vi "Process Trainer.vi"() -> ()   [LabVIEW 2019]
uses:
  <vilib>/Modbus/slave/Create Slave Instance (TCP).vi
  <vilib>/Modbus/slave/Modbus Slave.lvclass
panel:
  out "Waveform Graph":sgl[](graph)
  out "Hot water":sgl
  out "L1":sgl
  out "F2":sgl
  out "F1":sgl
  out "T3":sgl
  out "T2":sgl
  out "T1":sgl
  in  "Hot Water Setpoint":sgl(slide) scale=0.0..200.0
  in  "FV4":sgl(slide) scale=0.0..100.0
  in  "FV3":sgl(slide) scale=0.0..100.0
  in  "FV2":sgl(slide) scale=0.0..100.0
  in  "FV1":sgl(slide) scale=0.0..100.0
  in  "M2":sgl(slide) scale=0.0..100.0
  out "Hot Water Temp":sgl(knob) scale=0.0..100.0
  out "L1":sgl(knob) scale=0.0..100.0
  out "F2":sgl(knob) scale=0.0..100.0
  out "F1":sgl(knob) scale=0.0..100.0
  out "T3":sgl(knob) scale=0.0..100.0
  out "T2":sgl(knob) scale=0.0..100.0
  in  "stop":bool
  in  "M1":sgl(slide) scale=0.0..100.0
  out "T1":sgl(knob) scale=0.0..100.0
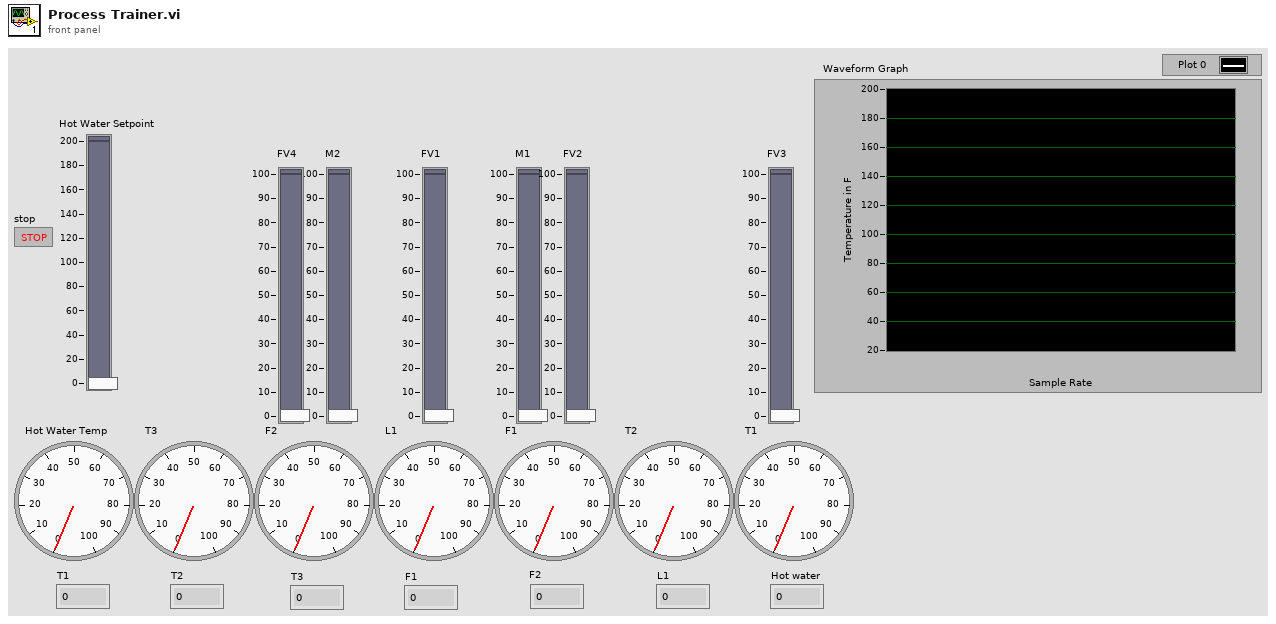
[diagram p1: front panel]
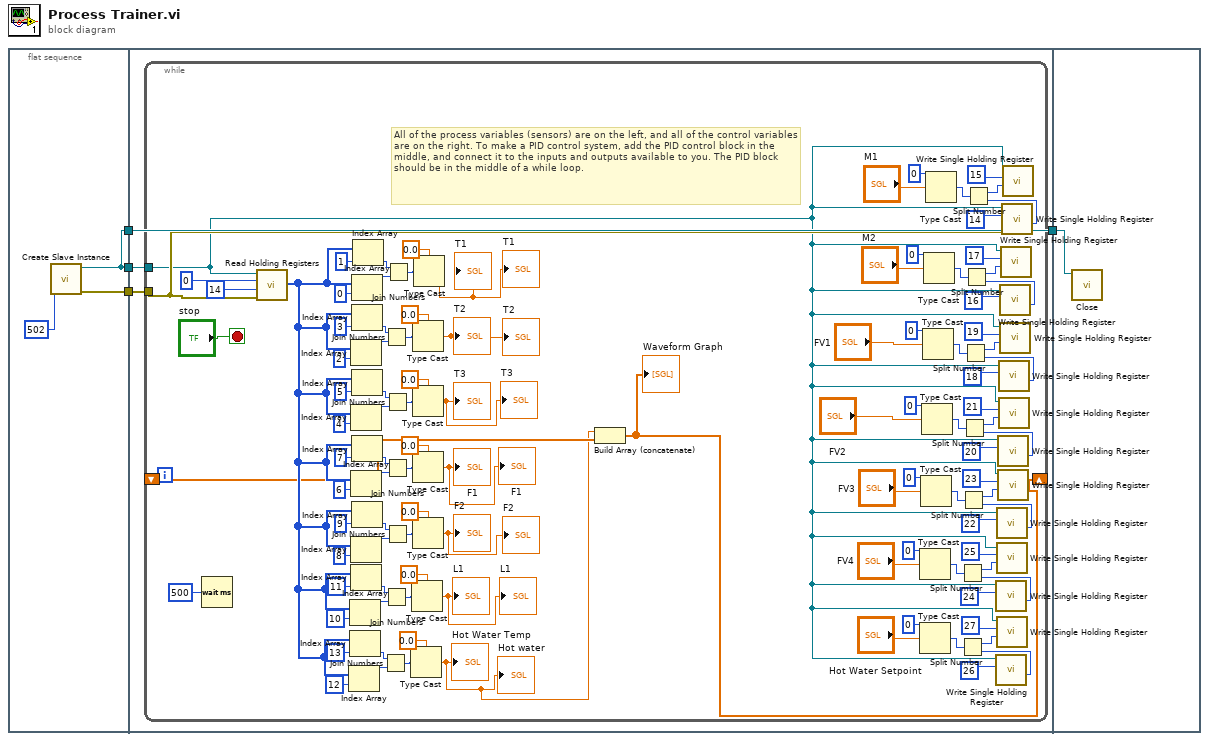
[diagram p0: block diagram]
diagram:
  n1 = flat-sequence {
    tunnel: [w5] -> w4
    tunnel: [w6] -> w3
    tunnel: [w5] -> w2
    tunnel: w4 -> [w10]
    tunnel: w3 -> [w9]
    tunnel: [w8] -> w1
    tunnel: w2 -> [w8]
    tunnel: w1 -> [w118]
    frame #0 {
      n2 = call-poly <vilib>:"Create Slave Instance.vi"("port (502)"=u16 502) -> ("error out"=w6:errorcluster, "TCP slave instance"=w5:refnum<class "Modbus Slave.lvclass">)  [unwired: 9 in]
    }
    frame #1 {
      n3 = while {
        tunnel: w10 -> [w21]
        tunnel: w9 -> [w113]
        shift-right: [w11] -> _
        shift-left: _ -> [w14]
        stop <- "stop" stop-if-true
        # "All of the process variables (sensors) are on the left, and all of the control variables are on the right. To make a PID control system, add the PID control block in the middle, and connect it to the inputs and outputs available to you. The PID block should be in the middle of a while loop."
        n4 = Wait (ms)(milliseconds to wait=u32 500) -> ()  [unwired: 1 out]
        n5 = call-dynamic "Read Holding Registers.vi"("error in (no error)"=w113, "number of holding registers"=u16 14, "starting address"=u16 0, "Modbus slave in"=w21) -> ("register values"=w64:u16[])  [unwired: 5 in, 2 out]
        n6 = Index Array(array=w64, index=12) -> (element=w66:u16)
        n7 = Index Array(array=w64, index=10) -> (element=w72:u16)
        n8 = Index Array(array=w64, index=13) -> (element=w65:u16)
        n9 = Index Array(array=w64, index=2) -> (element=w96:u16)
        n10 = Index Array(array=w64, index=4) -> (element=w90:u16)
        n11 = Index Array(array=w64, index=6) -> (element=w84:u16)
        n12 = Index Array(array=w64, index=8) -> (element=w78:u16)
        n13 = Index Array(array=w64, index=11) -> (element=w71:u16)
        n14 = Index Array(array=w64, index=0) -> (element=w102:u16)
        n15 = Index Array(array=w64, index=3) -> (element=w95:u16)
        n16 = Index Array(array=w64, index=5) -> (element=w89:u16)
        n17 = Index Array(array=w64, index=7) -> (element=w83:u16)
        n18 = Index Array(array=w64, index=9) -> (element=w77:u16)
        n19 = Index Array(array=w64, index=1) -> (element=w101:u16)
        n20 = Join Numbers(hi=w65, lo=w66) -> ((hi.lo)=w67:u32)
        n21 = Join Numbers(hi=w95, lo=w96) -> ((hi.lo)=w97:u32)
        n22 = Join Numbers(hi=w71, lo=w72) -> ((hi.lo)=w73:u32)
        n23 = Join Numbers(hi=w89, lo=w90) -> ((hi.lo)=w91:u32)
        n24 = Join Numbers(hi=w83, lo=w84) -> ((hi.lo)=w85:u32)
        n25 = Join Numbers(hi=w77, lo=w78) -> ((hi.lo)=w79:u32)
        n26 = Join Numbers(hi=w101, lo=w102) -> ((hi.lo)=w103:u32)
        n27 = Type Cast(type=sgl 0.0, x=w67) -> (*(type *) &x=w13:sgl)
        "Hot Water Temp" <- w13
        "Hot water" <- w13
        n28 = Type Cast(type=sgl 0.0, x=w73) -> (*(type *) &x=→"L1" →"L1":sgl)
        n29 = Type Cast(type=sgl 0.0, x=w97) -> (*(type *) &x=→"T2" →"T2":sgl)
        n30 = Type Cast(type=sgl 0.0, x=w91) -> (*(type *) &x=→"T3" →"T3":sgl)
        n31 = Type Cast(type=sgl 0.0, x=w85) -> (*(type *) &x=→"F1" →"F1":sgl)
        n32 = Type Cast(type=sgl 0.0, x=w79) -> (*(type *) &x=→"F2" →"F2":sgl)
        n33 = Type Cast(type=sgl 0.0, x=w103) -> (*(type *) &x=→"T1" →"T1":sgl)
        n34 = Build Array (concatenate)(w13, w14) -> (w11:sgl[])
        "Waveform Graph" <- w11
        n35 = Type Cast(type=u32 0, x="FV4") -> (*(type *) &x=w31:u32)
        n36 = Type Cast(type=u32 0, x="Hot Water Setpoint") -> (*(type *) &x=w24:u32)
        n37 = Type Cast(type=u32 0, x="FV3") -> (*(type *) &x=w38:u32)
        n38 = Type Cast(type=u32 0, x="FV2") -> (*(type *) &x=w45:u32)
        n39 = Type Cast(type=u32 0, x="FV1") -> (*(type *) &x=w52:u32)
        n40 = Type Cast(type=u32 0, x="M2") -> (*(type *) &x=w59:u32)
        n41 = Type Cast(type=u32 0, x="M1") -> (*(type *) &x=w109:u32)
        n42 = Split Number(x=w31) -> (hi(x)=w33:u16, lo(x)=w32:u16)
        n43 = Split Number(x=w24) -> (hi(x)=w26:u16, lo(x)=w25:u16)
        n44 = Split Number(x=w38) -> (hi(x)=w40:u16, lo(x)=w39:u16)
        n45 = Split Number(x=w45) -> (hi(x)=w47:u16, lo(x)=w46:u16)
        n46 = Split Number(x=w52) -> (hi(x)=w54:u16, lo(x)=w53:u16)
        n47 = Split Number(x=w59) -> (hi(x)=w61:u16, lo(x)=w60:u16)
        n48 = Split Number(x=w109) -> (hi(x)=w111:u16, lo(x)=w110:u16)
        n49 = call-dynamic "Write Single Holding Register.vi"("holding register value"=w32, "address"=u16 24, "Modbus slave in"=w21) -> ()  [unwired: 7 in, 2 out]
        n50 = call-dynamic "Write Single Holding Register.vi"("holding register value"=w25, "address"=u16 26, "Modbus slave in"=w21) -> ()  [unwired: 7 in, 2 out]
        n51 = call-dynamic "Write Single Holding Register.vi"("holding register value"=w39, "address"=u16 22, "Modbus slave in"=w21) -> ()  [unwired: 7 in, 2 out]
        n52 = call-dynamic "Write Single Holding Register.vi"("holding register value"=w33, "address"=u16 25, "Modbus slave in"=w21) -> ()  [unwired: 7 in, 2 out]
        n53 = call-dynamic "Write Single Holding Register.vi"("holding register value"=w26, "address"=u16 27, "Modbus slave in"=w21) -> ()  [unwired: 7 in, 2 out]
        n54 = call-dynamic "Write Single Holding Register.vi"("holding register value"=w46, "address"=u16 20, "Modbus slave in"=w21) -> ()  [unwired: 7 in, 2 out]
        n55 = call-dynamic "Write Single Holding Register.vi"("holding register value"=w40, "address"=u16 23, "Modbus slave in"=w21) -> ()  [unwired: 7 in, 2 out]
        n56 = call-dynamic "Write Single Holding Register.vi"("holding register value"=w53, "address"=u16 18, "Modbus slave in"=w21) -> ()  [unwired: 7 in, 2 out]
        n57 = call-dynamic "Write Single Holding Register.vi"("holding register value"=w47, "address"=u16 21, "Modbus slave in"=w21) -> ()  [unwired: 7 in, 2 out]
        n58 = call-dynamic "Write Single Holding Register.vi"("holding register value"=w60, "address"=u16 16, "Modbus slave in"=w21) -> ()  [unwired: 7 in, 2 out]
        n59 = call-dynamic "Write Single Holding Register.vi"("holding register value"=w54, "address"=u16 19, "Modbus slave in"=w21) -> ()  [unwired: 7 in, 2 out]
        n60 = call-dynamic "Write Single Holding Register.vi"("holding register value"=w61, "address"=u16 17, "Modbus slave in"=w21) -> ()  [unwired: 7 in, 2 out]
        n61 = call-dynamic "Write Single Holding Register.vi"("error in (no error)"=w113, "holding register value"=w110, "address"=u16 14, "Modbus slave in"=w21) -> ()  [unwired: 6 in, 2 out]
        n62 = call-dynamic "Write Single Holding Register.vi"("holding register value"=w111, "address"=u16 15, "Modbus slave in"=w21) -> ()  [unwired: 7 in, 2 out]
      }
    }
    frame #2 {
      n63 = call-dynamic "Close.vi"("Modbus slave in"=w118) -> ()  [unwired: 10 in, 1 out]
    }
  }
